vi "Reverse waveform.vi"(10 "Waveform":waveform(dbl)) -> (2 "Output Waveform":waveform(dbl))   [LabVIEW 2015]
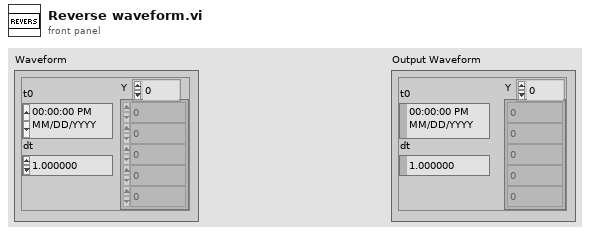
[diagram p1: front panel]
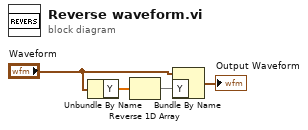
[diagram p0: block diagram]
diagram:
  n1 = Unbundle By Name("Waveform") -> ("Y"=w4:dbl[])
  n2 = Reverse 1D Array(array=w4) -> (reversed array=w3:dbl[])
  n3 = Bundle By Name(cluster="Waveform", "Y"=w3) -> (→"Output Waveform":waveform(dbl))
